vi "RT_stage_control_step_response_rev2.vi"() -> ()   [LabVIEW 2019]
uses:
  <vilib>/Platform/TimedLoop/XDataNode/timing_clust.ctl
  <vilib>/Platform/TimedLoop/XDataNode/nitl_modes.ctl
  <vilib>/Platform/TimedLoop/XDataNode/wakeup.ctl
  <vilib>/FPGAPlugInAG/myRIO-1900/niLvFpga_Open_myRIO-1900.vi
  <vilib>/rvi/interface/common/dynamic/niFpgaDynamicAddResources.vi
  <vilib>/Utility/error.llb/Error Cluster From Error Code.vi
  <vilib>/rvi/errors/niLvFpgaAdjustHostInterfaceError.vi
  <vilib>/rvi/interface/nirviOpenFPGA/nirviOpenFPGA.xnode
  FPGA Bitfiles/studentchallenge_FPGATarget_FPGARADCWDAC3_gNVwU-DQYMc.lvbitx
  FPGA_R_ADC_W_DAC.vi
  <vilib>/Platform/TimedLoop/XDataNode/XDataNode.xnode
  <vilib>/rvi/interface/nirviReadWriteControl/nirviReadWriteControl.xnode
  <vilib>/Platform/TimedLoop/XDataNode/XDNodeRunTimeDep.lvlib
  NiFpgaLv.dll
  <vilib>/rvi/interface/Simulation/niFpgaSimulationCallBeginRW.vi
panel:
  out "N late finishes":i32
  in  "integral  reset":bool
  in  "D":dbl=1000.0
  in  "desired position (mm)":dbl step=0.008 format="%_6g"
  out "Finished Late? [i-1]":bool
  in  "windup-":dbl=-2.0
  in  "windup +":dbl=2.0
  in  "manual":dbl=-0.8009999999999999 step=0.03 format="%_6g"
  in  "PID control":bool
  in  "lower limit":dbl=-1.0
  in  "upper limit":dbl=0.1
  in  "I":dbl=0.01 format="%#_6f"
  in  "P":dbl=5.0 format="%#_6f"
  in  "stop":bool
  in  "ADC Select":u16(ring)=32 items=["ADC 1"=32, "ADC 2"=40, "ADC 3"=36, "ADC 4"=44]
  in  "Reset Sensors":bool
  out "Displacement (mm)":cluster{dbl, dbl, "upper limit":dbl}(graph)
  # "CAP PROBE"
  # "ENCODER"
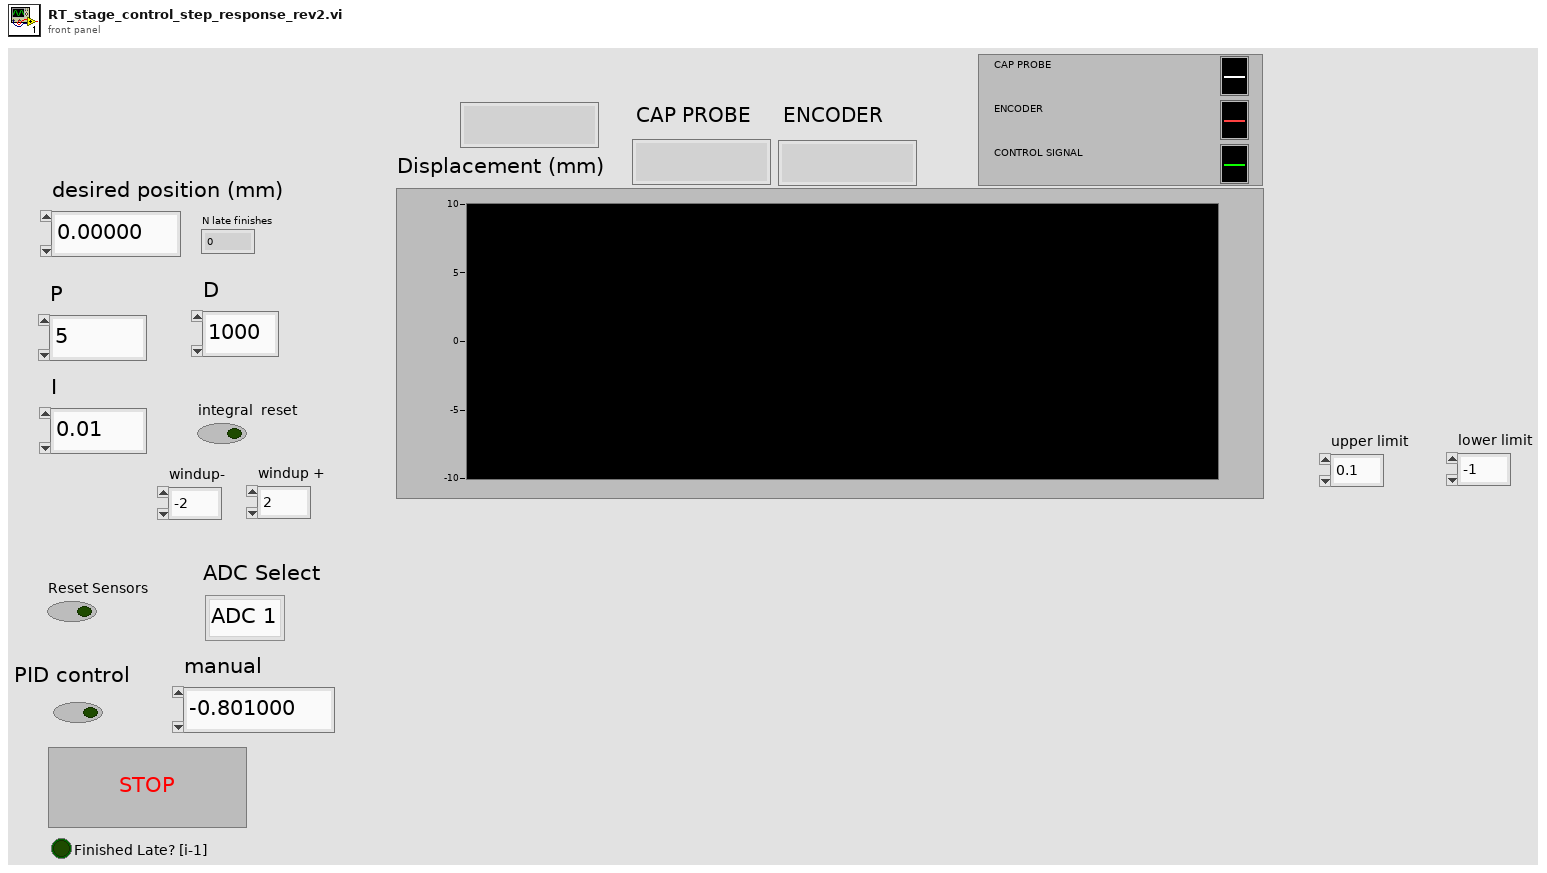
[diagram p1: front panel]
types:
  T1 = typedef "XDNodeRunTimeDep.lvlib/timing_clust.ctl" = cluster{"Expected End [f-1]":u64, "Actual End [f-1]":u64, "Finished Late? [f-1]":bool, "Expected End [i-1]":u64, "Actual End [i-1]":u64, "Finished Late? [i-1]":bool, "Expected Start [i]":u64, "Actual Start [i]":u64, "Expected Start [f]":u64, "Actual Start [f]":u64, "Source Name":string, "Structure Name":string, "Period":i64, "Deadline":i64, "Offset":i64, "Start":i64, "Priority":i32, "Timeout":i32, "Mode":T2, "Wakeup Reason":T3, "Error":errorcluster, "Source Type":string, "Secondary Source Type":string, "Global End Time":u64, "Global Start Time":u64, "Frame Duration":u64, "Iteration Duration":u64, "Assigned CPU":i32, "I/O Scan Engine Mode":u32}
  T2 = typedef "XDNodeRunTimeDep.lvlib/nitl_modes.ctl" = enum32{"No Change", "Process missed periods, maintain original phase", "Discard missed periods, maintain original phase", "Process missed periods, ignore original phase", "Discard missed periods, ignore original phase"}
  T3 = typedef "XDNodeRunTimeDep.lvlib/wakeup.ctl" = enum32{"Normal", "Aborted", "Asynchronous wakeup", "Timing source error", "Timed loop error", "Timeout"}
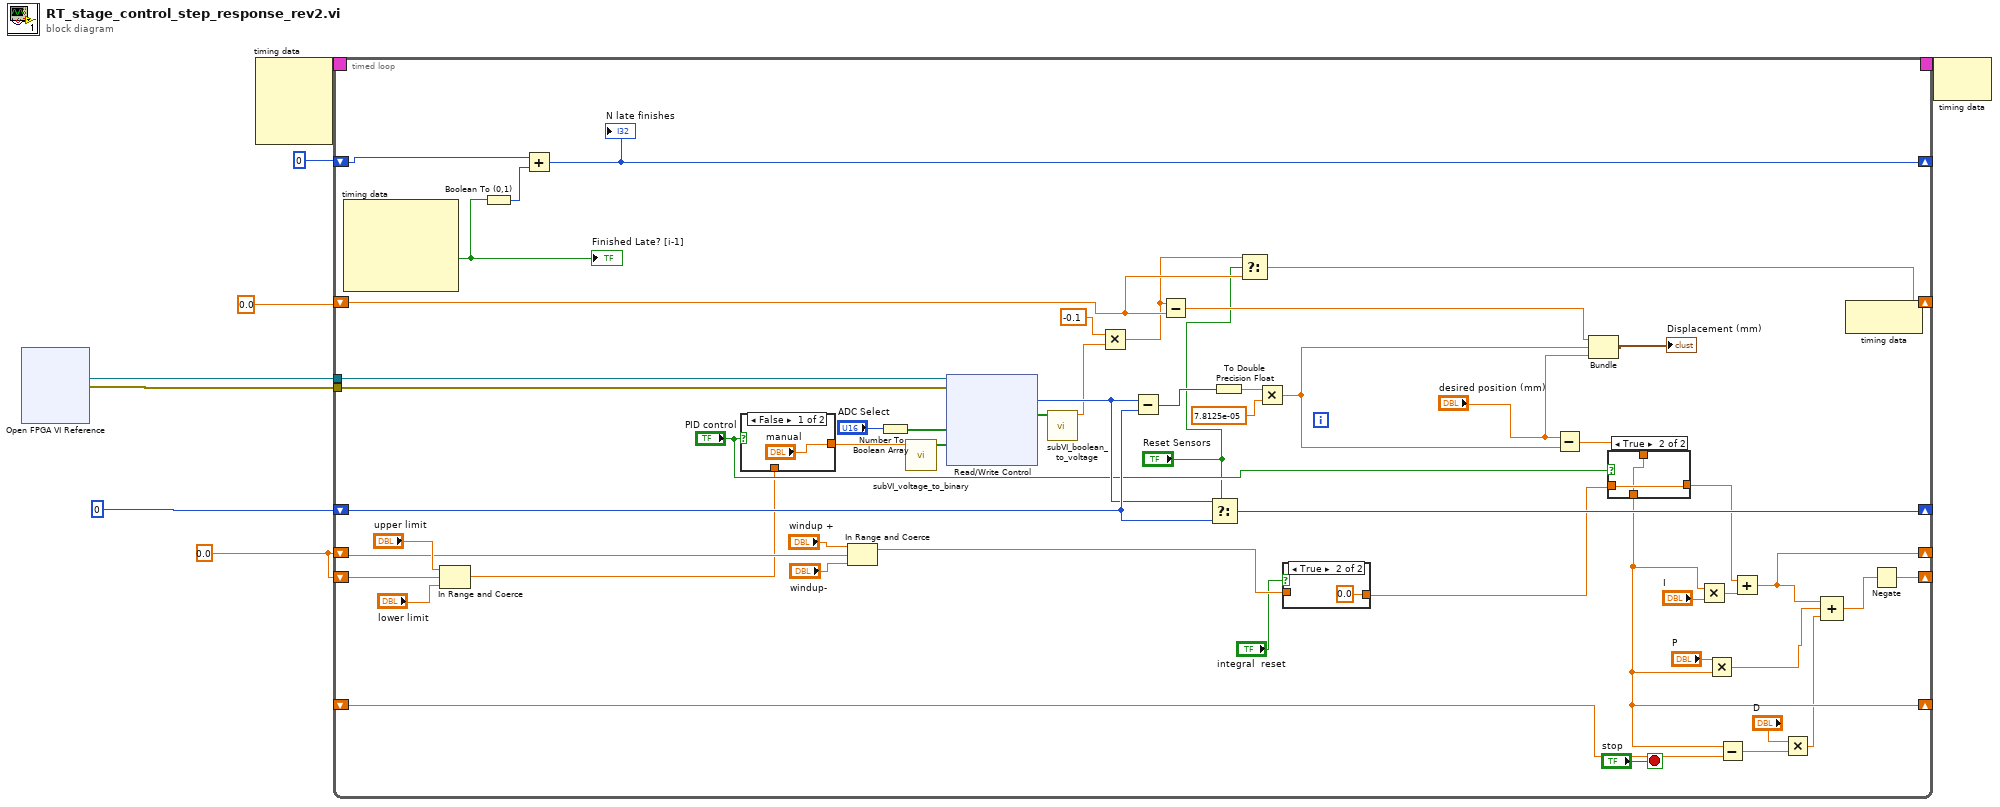
[diagram p0: block diagram]
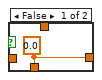
[diagram p3: hidden frame]
diagram:
  w3 = 0.0
  n1 = xnode "Open FPGA VI Reference"() -> ("FPGA VI Reference Out"=w8:refnum<k20>, "error out"=w6:errorcluster)  [unwired: 2 in]
  n2 = node-c288() -> (w5:T1)  [unwired: 4 in]
  n3 = timed-loop {
    tunnel: w8 -> [w61]
    shift-right: [w58] -> _
    shift-left: 0 -> [w56]
    tunnel: w6 -> [w52]
    shift-right: [w13] -> _
    shift-left: w3 -> [w47]
    timing: w5 -> [_]
    timing-out: [_] -> w4
    shift-right: [w34] -> _
    shift-left: w3 -> [w41]
    shift-right: [w38] -> _
    shift-left: _ -> [w37]
    shift-right: [w22] -> _
    shift-left: 0.0 ("x") -> [w21]
    shift-right: [w14] -> _
    shift-left: 0 -> [w15]
    stop <- "stop" stop-if-true
    n4 = node-c288() -> (w17:bool)  [unwired: 1 in, 4 out]
    "Finished Late? [i-1]" <- w17
    n5 = In Range and Coerce(upper limit="upper limit", x=w47, lower limit="lower limit") -> (coerced(x)=w11:dbl)  [unwired: 1 out]
    n6 = Boolean To (0,1)(Boolean=w17) -> (0, 1=w16:i16)
    n7 = Add(x=w15, y=w16) -> (x+y=w14:i32)
    "N late finishes" <- w14
    n8 = case shown="False" "PID control" {
      tunnel: ["manual" w68] -> w31
      tunnel: w11 -> [_ w68]
      frame False {
      }
      frame True {
      }
    }
    n9 = In Range and Coerce(upper limit="windup +", x=w41, lower limit="windup-") -> (coerced(x)=w30:dbl)  [unwired: 1 out]
    n10 = Number To Boolean Array(number="ADC Select") -> (Boolean array=w54:bool[])
    n11 = call "subVI_voltage_to_binary.vi"("voltage"=w31) -> ("binary"=w53:bool[])  [unwired: 10 in]
    n12 = xnode "Read/Write Control"("FPGA VI Reference In"=w61, "error in"=w52, "ADC write"=w54, "DAC 1 write"=w53) -> ("Encoder A"=w48:i32, "ADC read"=w26:bool[])  [unwired: 3 out]
    n13 = call "subVI_boolean_to_voltage.vi"("ADC read"=w26) -> ("V"=w24:dbl)  [unwired: 10 in]
    n14 = Multiply(x=-0.1, y=w24) -> (x*y=w18:dbl)
    n15 = Subtract(x=w48, y=w56) -> (x-y=w57:i32)
    n16 = Subtract(x=w18, y=w21) -> (x-y=w20:dbl)
    n17 = Select(t=w48, s="Reset Sensors", f=w56) -> (s? t:f=w58:i32)
    n18 = To Double Precision Float(number=w57) -> (double precision float=w59:dbl)
    n19 = Select(t=w18, s="Reset Sensors", f=w21) -> (s? t:f=w22:dbl)
    n20 = Multiply(x=w59, y=7.8125e-05) -> (x*y=w25:dbl)
    n21 = case shown="True" "integral  reset" {
      tunnel: [w62 0.0] -> w29
      tunnel: w30 -> [w62 _]
      frame False {
      }
      frame True {
      }
    }
    n22 = Subtract(x="desired position (mm)", y=w25) -> (x-y=w27:dbl)
    n23 = Bundle(w20, w25, "desired position (mm)"="desired position (mm)") -> (→"Displacement (mm)":cluster{dbl, dbl, "desired position (mm)":dbl})  [unwired: 1 in]
    n24 = case shown="True" "PID control" {
      tunnel: w29 -> [_ w66]
      tunnel: [w64 w66] -> w42
      tunnel: w27 -> [_ w65]
      tunnel: [w64 w65] -> w38
      frame False {
        w64 = 0.0
      }
      frame True {
      }
    }
    n25 = Multiply(x=w38, y="I") -> (x*y=w46:dbl)
    n26 = Multiply(x="P", y=w38) -> (x*y=w33:dbl)
    n27 = Subtract(x=w38, y=w37) -> (x-y=w36:dbl)
    n28 = Add(x=w42, y=w46) -> (x+y=w34:dbl)
    n29 = Multiply(x="D", y=w36) -> (x*y=w32:dbl)
    n30 = Compound Arithmetic op=ADD(w34, w33, w32) -> (w12:dbl)
    n31 = node-c288() -> ()  [unwired: 1 in, 1 out]
    n32 = Negate(x=w12) -> (-x=w13:dbl)
  }
  n33 = node-c288(w4) -> ()  [unwired: 1 out]
